vi "Resource Casting.vi"(8 "error in (no error)":errorcluster, 10 "VISA Resource In":refnum<visa-resource-name>, 11 "PXIe5105 in":refnum<class "PXIe5105.lvclass">) -> (0 "error out":errorcluster, 2 "Resource String":string, 3 "PXIe5105 out":refnum<class "PXIe5105.lvclass">)   [LabVIEW 2018, in "PXIe5105.lvlib" / "PXIe5105.lvclass"]
uses:
  PXIe5105.lvclass
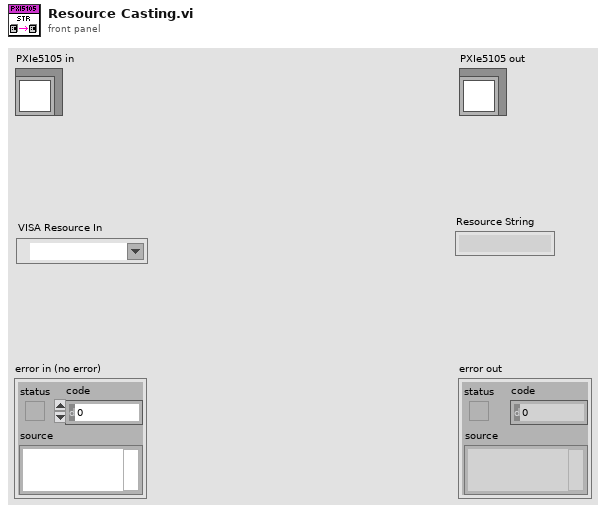
[diagram p1: front panel]
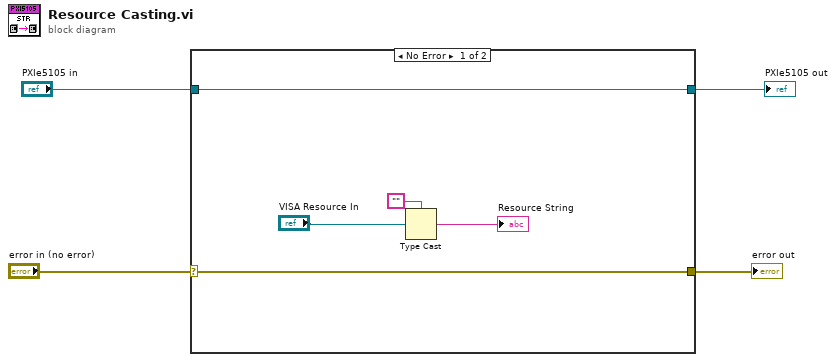
[diagram p0: block diagram]
diagram:
  n1 = case shown="No Error" "error in (no error)" {
    selector: "error in (no error)" -> [w8 w11]
    tunnel: [w8 w11] -> w3
    tunnel: [w9 w10] -> w1
    tunnel: "PXIe5105 in" -> [w9 w10]
    frame No Error {
      n2 = Type Cast(type="", x="VISA Resource In") -> (*(type *) &x=→"Resource String":string)
    }
    frame Error {
    }
  }
  "error out" <- w3
  "PXIe5105 out" <- w1
